vi "EnterFlujos S-F.vi"(6 "error in (no error)":errorcluster, 7 "FLOWBUS MassFlowDevs":T1, 8 "SERIAL MassFlowDevs":T1) -> (0 "error out":errorcluster, 1 "%MFCf":dbl[](array[numeric]) format="%.1g", 2 "%MFCs":dbl[](array[numeric]) format="%.1g", 3 "Cancelled?":bool)   [LabVIEW 2013]
doc: "Use this template to create a dialog box. This template polls the state of the buttons on the front panel and does not use events. Use the Dialog Using Events template (not available in Base package) to create a dialog box with event handling."
uses:
  serialBronkhorst/_s_TablaBronkhorst.ctl
panel:
  in  "SP4 2":dbl format="%.2f"
  in  "SP3 2":dbl format="%.2f"
  in  "SP2 2":dbl format="%.2f"
  in  "SP1 2":dbl format="%.2f"
  in  "SP4":dbl format="%.2f"
  in  "SP3":dbl format="%.2f"
  in  "SP2":dbl format="%.2f"
  in  "SP1":dbl format="%.2f"
  in  "Cancel":bool
  in  "OK":bool
  # "Flujos de gases y líquidos:"
  # "NUEVO"
  # "NUEVO"
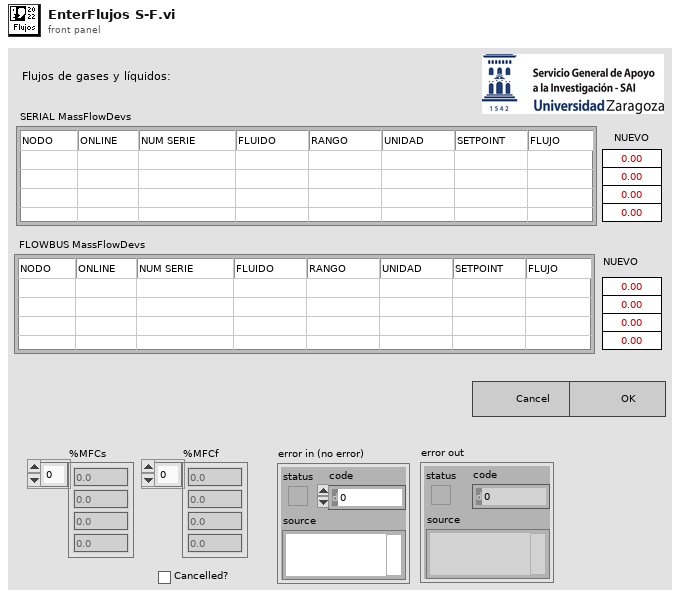
[diagram p1: front panel]
types:
  T1 = typedef "_s_TablaBronkhorst.ctl" = string[][]
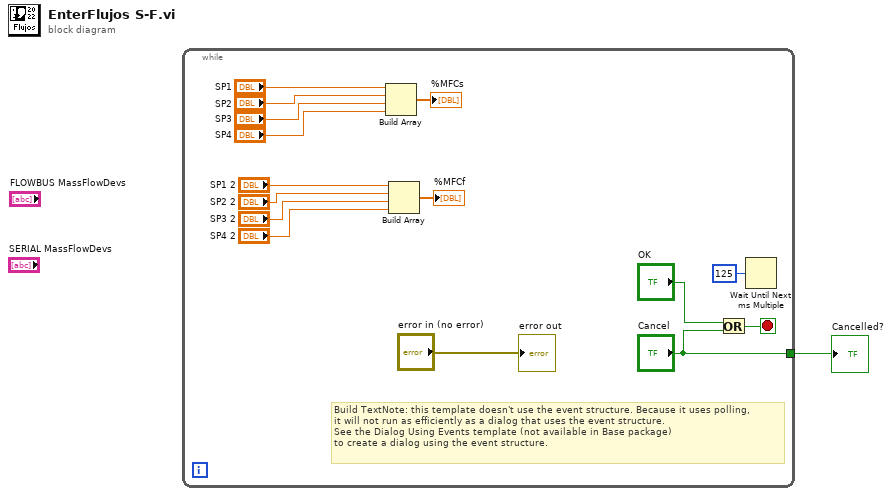
[diagram p0: block diagram]
diagram:
  n1 = while {
    tunnel: ["Cancel"] -> w1
    stop <- w15 stop-if-true
    # "Build TextNote: this template doesn't use the event structure. Because it uses polling, \nit will not run as efficiently as a dialog that uses the event structure.\nSee the Dialog Using Events template (not available in Base package) \nto create a dialog using the event structure."
    n2 = Build Array("SP1", "SP2", "SP3", "SP4") -> (→"%MFCs":dbl[])
    n3 = Build Array("SP1 2", "SP2 2", "SP3 2", "SP4 2") -> (→"%MFCf":dbl[])
    n4 = Or(x="OK", y="Cancel") -> (x .or. y?=w15:bool)
    n5 = Wait Until Next ms Multiple(millisecond multiple=u32 125) -> ()  [unwired: 1 out]
    "error out" <- "error in (no error)"
  }
  "Cancelled?" <- w1
